vi "Read UI Configuration Information.vi"(8 "error in (no error)":errorcluster, 11 "UI Initialize in":refnum<class "UI Initialize.lvclass">) -> (0 "error out":errorcluster, 2 "UI Configuration Information":T1={"Space Between Buttons"=3, "Number of Buttons to Show"=6, "Header Image"=path "Images/Blue Background.bmp", "Footer Image"=path "Images/Blue Background.bmp"}, 3 "UI Initialize out":refnum<class "UI Initialize.lvclass">)   [LabVIEW 2011, in "UI Initialize.lvclass"]
uses:
  UI Initialize.lvclass
  UI Control Definitions/UI Configuration Information.ctl
  UI Initialize.lvclass/UI Initialize.ctl
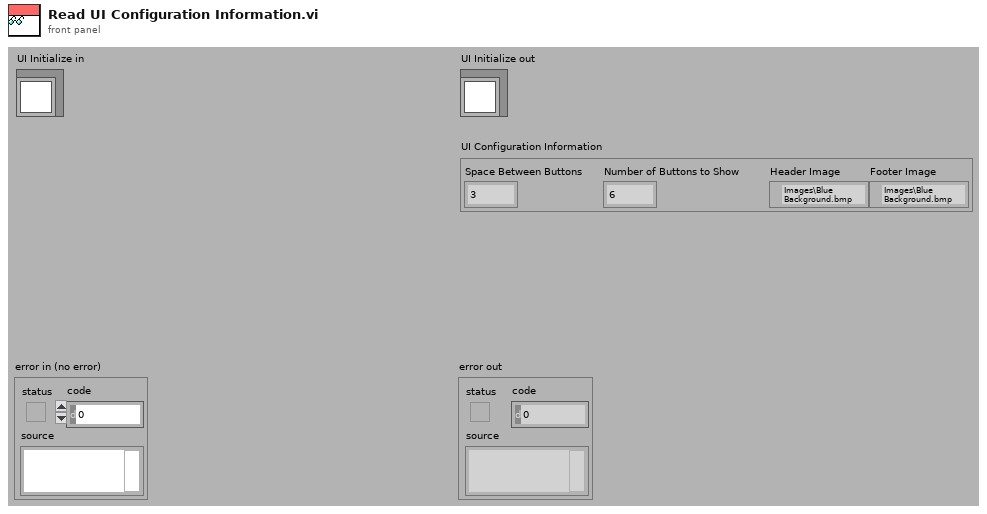
[diagram p1: front panel]
types:
  T1 = typedef "UI Configuration Information.ctl" = cluster{"Space Between Buttons":i32, "Number of Buttons to Show":i32, "Header Image":path, "Footer Image":path}
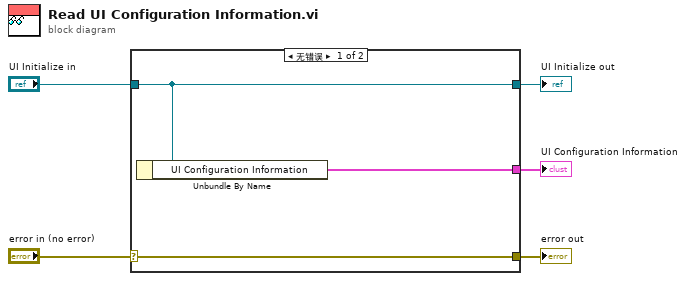
[diagram p0: block diagram]
diagram:
  n1 = case shown="无错误" "error in (no error)" {
    selector: "error in (no error)" -> [w8 w9]
    tunnel: [w8 w9] -> w4
    tunnel: [w7 w10] -> w2
    tunnel: "UI Initialize in" -> [w7 w10]
    tunnel: [w6 _] -> w1
    frame No Error {
      n2 = Unbundle By Name(w7) -> ("UI Configuration Information"=w6:T1)
    }
    frame Error {
    }
  }
  "error out" <- w4
  "UI Initialize out" <- w2
  "UI Configuration Information" <- w1
